vi "数据查询_数据查询_古田户外.vi"() -> ()   [LabVIEW 2016]
uses:
  <vilib>/Utility/miscctls.llb/LVPointTypeDef.ctl
  <vilib>/Utility/miscctls.llb/LVRowAndColumnUnsignedTypeDef.ctl
  <vilib>/addons/database/_DB Variant To Data/Database Variant To Data.xnode
panel:
  in  "工作模式":string(combo)="全部数据"
  out "连接的字符串":string
  out "选中数据表":string
  in  "查询":bool
  in  "结束日期":string="2020/01/01"
  in  "起始日期":string="2010/01/01"
  out "XY图":cluster{"data":timestamp[], "data":dbl[]}[](graph)
  in  "组合框":string(combo)
  out "数据表":string[][](table)
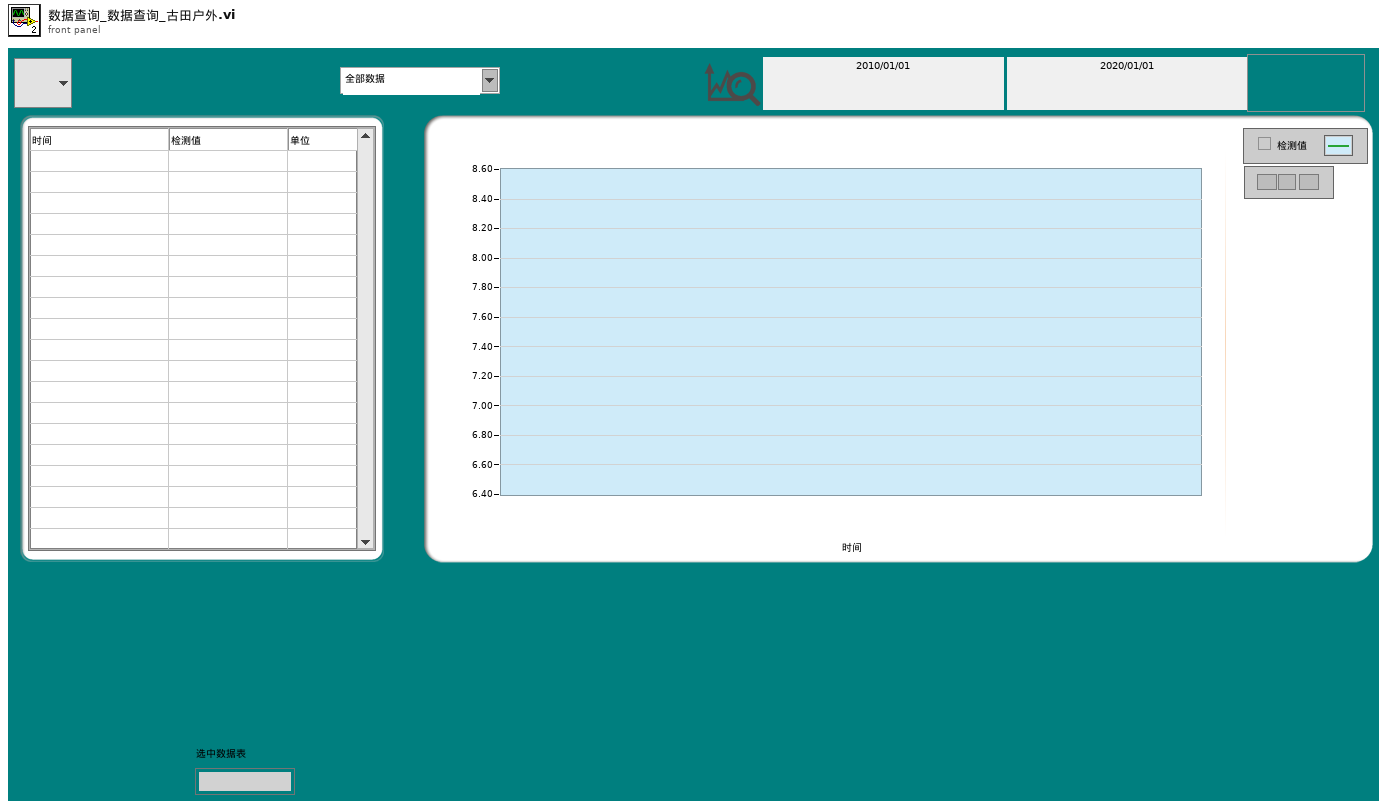
[diagram p1: front panel]
types:
  T1 = typedef "LVPointTypeDef.ctl" = cluster{"Horizontal":i16, "Vertical":i16}
  T2 = typedef "LVRowAndColumnUnsignedTypeDef.ctl" = cluster{"Row":u32, "Column":u32}
  T3 = typedef "LVPoint32TypeDef.ctl" = cluster{"Horizontal":i32, "Vertical":i32}
  T4 = typedef "LVPointDoubleTypeDef.ctl" = cluster{"Cursor X":dbl, "Cursor Y":dbl}
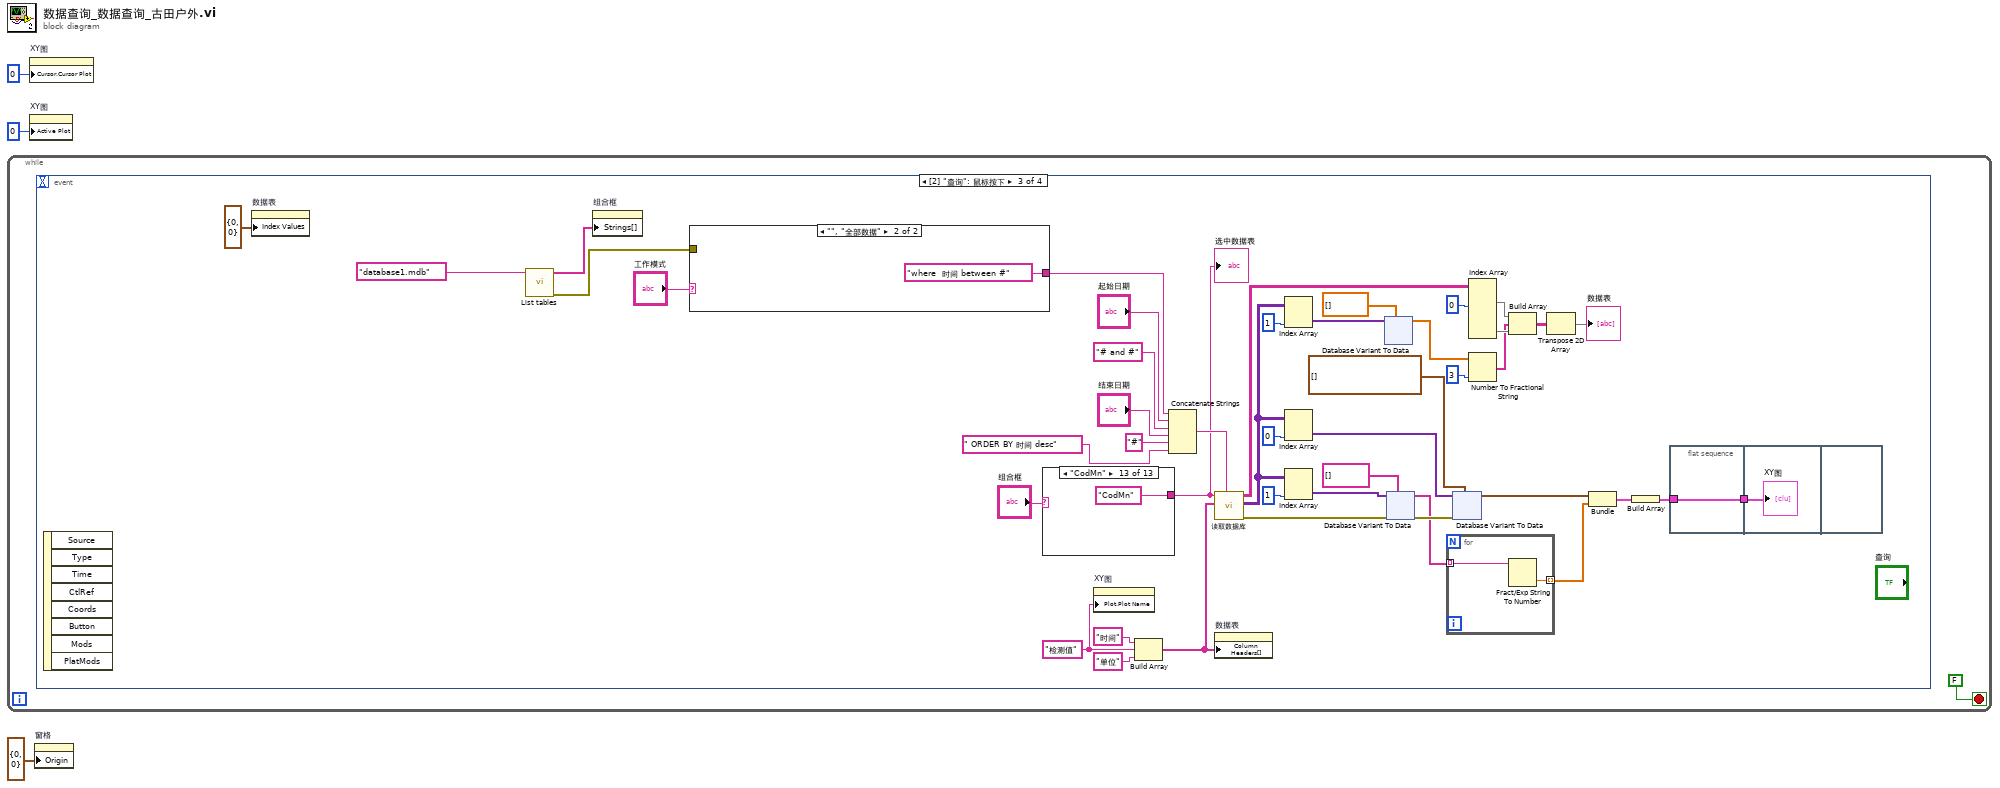
[diagram p0: block diagram]
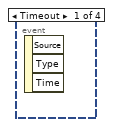
[diagram p2: hidden frame]
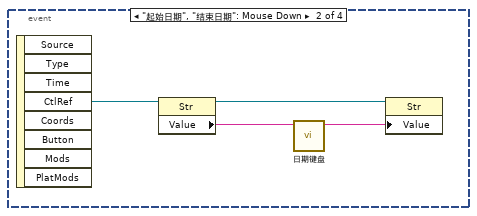
[diagram p3: hidden frame]
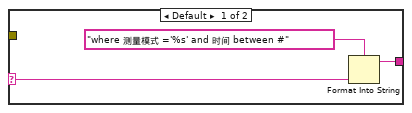
[diagram p4: hidden frame]
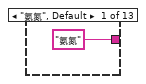
[diagram p5: hidden frame]
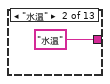
[diagram p6: hidden frame]
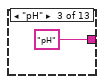
[diagram p7: hidden frame]
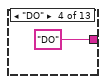
[diagram p8: hidden frame]
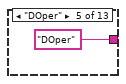
[diagram p9: hidden frame]
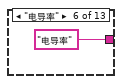
[diagram p10: hidden frame]
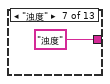
[diagram p11: hidden frame]
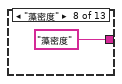
[diagram p12: hidden frame]
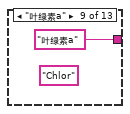
[diagram p13: hidden frame]
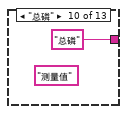
[diagram p14: hidden frame]
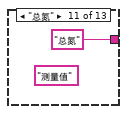
[diagram p15: hidden frame]
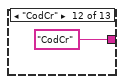
[diagram p16: hidden frame]
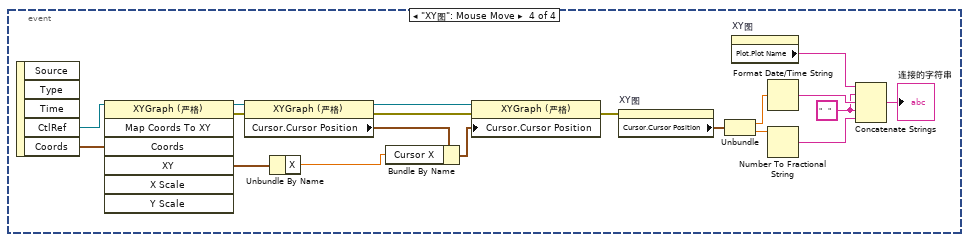
[diagram p17: hidden frame]
diagram:
  n1 = while {
    stop <- FALSE stop-if-true
    n2 = event shown="[2] \"查询\": 鼠标按下" {
      selector: _ -> [_ _ _ _]
      dyn-events: _ -> [_ _ _ _]
      timeout: _ -> [_ _ _ _]
      event Timeout {
        n3 = event-data() -> ()  [unwired: 1 in, 3 out]
      }
      event "起始日期", "结束日期": Mouse Down {
        n4 = event-data() -> ("CtlRef"=w8:refnum<vi>)  [unwired: 1 in, 7 out]
        n5 = property class="Str"(reference=w8) -> (reference out=w6:refnum<vi>, "Value"=w7:string)  [unwired: 1 in, 1 out]
        n6 = call "日期键盘.vi"("原值"=w7) -> ("x+y"=w5:string)  [unwired: 10 in]
        n7 = property class="Str"(reference=w6, "Value"=w5) -> ()  [unwired: 1 in, 2 out]
      }
      event "查询": Mouse Down {
        w25 = "检测值"
        n8 = event-data() -> ()  [unwired: 1 in, 8 out]
        n9 = property on="数据表" class="Tbl (严格)"("Index Values"=T2 {"Row"=0, "Column"=0} ("索引值")) -> ()  [unwired: 2 in, 2 out]
        n10 = call "List tables.vi"("database"="database1.mdb") -> ("error out"=w9:errorcluster, "tables"=w10:string[])  [unwired: 9 in]
        n11 = property on="组合框" class="CmbBox"("Strings[]"=w10) -> ()  [unwired: 2 in, 2 out]
        n12 = case shown="\"\", \"全部数据\"" "工作模式" {
          selector: "工作模式" -> [w56 _]
          tunnel: [w54 "where  时间 between #" ("condition")] -> w13
          tunnel: w9 -> [_ _]
          frame Default {
            n13 = Format Into String(format string="where 测量模式 ='%s' and 时间 between #" ("condition"), w56) -> (resulting string=w54:string)  [unwired: 2 in, 1 out]
          }
          frame "", "全部数据" {
          }
        }
        n14 = case shown="\"CodMn\"" "组合框" {
          tunnel: ["氨氮" "水温" "pH" "DO" "DOper" "电导率" "浊度" "藻密度" "叶绿素a" "总磷" "总氮" "CodCr" "CodMn"] -> w27
          frame "氨氮", Default {
          }
          frame "水温" {
          }
          frame "pH" {
          }
          frame "DO" {
          }
          frame "DOper" {
          }
          frame "电导率" {
          }
          frame "浊度" {
          }
          frame "藻密度" {
          }
          frame "叶绿素a" {
            (unwired) "Chlor"
          }
          frame "总磷" {
            (unwired) "测量值"
          }
          frame "总氮" {
            (unwired) "测量值"
          }
          frame "CodCr" {
          }
          frame "CodMn" {
          }
        }
        "选中数据表" <- w27
        n15 = property on="XY图" class="XYGraph (严格)"("Plot.Plot Name"=w25) -> ()  [unwired: 2 in, 2 out]
        n16 = Build Array("时间", w25, "单位" ("元素")) -> (w28:string[])
        n17 = Concatenate Strings(w13, "起始日期", "# and #" ("condition"), "结束日期", "#" ("condition"), " ORDER BY 时间 desc" ("字符串")) -> (w52:string)
        n18 = call "读取数据库.vi"("condition"=w52, "显示项"=w28, "组合框"=w27) -> ("error out"=w43:errorcluster, "data"=w22:variant[][], "表格"=w35:string[][])  [unwired: 5 in, 1 out]
        n19 = property on="数据表" class="Tbl (严格)"("Column Headers[]"=w28) -> ()  [unwired: 2 in, 2 out]
        n20 = Index Array(array=w22, index (col)=1 ("禁用的索引 (列)")) -> (element=w20:variant[])  [unwired: 1 in]
        n21 = Index Array(array=w22, index (col)=0 ("禁用的索引 (列)")) -> (element=w46:variant[])  [unwired: 1 in]
        n22 = Index Array(array=w22, index (col)=1 ("禁用的索引 (列)")) -> (element=w44:variant[])  [unwired: 1 in]
        n23 = xnode "Database Variant To Data"("database variant"=w20, "type"=sgl[] []) -> ("data"=w18:sgl[])  [unwired: 1 in, 1 out]
        n24 = xnode "Database Variant To Data"("database variant"=w44, "error in (no error)"=w43, "type"=string[] []) -> ("data"=w26:string[], "error out"=w42:errorcluster)
        n25 = for {
          tunnel: w26 -> [w97] mode=indexing
          tunnel: [w96] -> w12 mode=indexing
          n26 = Fract/Exp String To Number(string=w97) -> (number=w96:dbl)  [unwired: 3 in, 1 out]
        }
        n27 = xnode "Database Variant To Data"("database variant"=w46, "error in (no error)"=w42, "type"=timestamp[] []) -> ("data"=w37:timestamp[])  [unwired: 1 out]
        n28 = Index Array(array=w35, index (col) #1=0 ("禁用的索引 (列)")) -> (element #1=w33:string[], element #3=w23:string[])  [unwired: 5 in, 1 out]
        n29 = Number To Fractional String(number=w18, precision (6)=i16 3 ("精度(6)")) -> (F-format string=w16:string[])  [unwired: 2 in]
        n30 = Build Array(w33, w16, w23) -> (w32:string[][])
        n31 = Transpose 2D Array(2D array=w32) -> (transposed array=→"数据表":string[][])
        n32 = Bundle("data"=w37, w12) -> (w38:cluster{"data":timestamp[], dbl[]})  [unwired: 1 in]
        n33 = Build Array(w38) -> (w39:cluster{"data":timestamp[], dbl[]}[])
        n34 = flat-sequence {
          tunnel: [w111] -> w40
          tunnel: w39 -> [w111]
          tunnel: w40 -> [w112]
          frame #0 {
          }
          frame #1 {
            "XY图" <- w112
          }
          frame #2 {
          }
        }
      }
      event "XY图": Mouse Move {
        w214 = "   " ("字符串")
        n35 = event-data() -> ("CtlRef"=w221:refnum<vi>, "Coords"=w220:T3)  [unwired: 1 in, 3 out]
        n36 = invoke class="XYGraph (严格)" method="Map Coords To XY"(reference=w221, "Coords"=w220) -> (reference out=w209:refnum<vi>, error out=w207:errorcluster, "XY"=w210:cluster{"X":dbl, "Y":dbl})  [unwired: 5 in, 4 out]
        n37 = property class="XYGraph (严格)"(reference=w209, error in=w207) -> (reference out=w208:refnum<vi>, error out=w206:errorcluster, "Cursor.Cursor Position"=w205:T4)
        n38 = Unbundle By Name(w210) -> ("X"=w204:dbl)
        n39 = Bundle By Name(cluster=w205, "Cursor X"=w204) -> (w203:T4)
        n40 = property class="XYGraph (严格)"(reference=w208, error in=w206, "Cursor.Cursor Position"=w203) -> (error out=w219:errorcluster)  [unwired: 1 out]
        n41 = property on="XY图" class="XYGraph (严格)"(error in=w219) -> ("Cursor.Cursor Position"=w217:T4)  [unwired: 1 in, 2 out]
        n42 = Unbundle(w217) -> ("Cursor X"=w216:dbl, "Cursor Y"=w213:dbl)
        n43 = property on="XY图" class="XYGraph (严格)"() -> ("Plot.Plot Name"=w211:string)  [unwired: 2 in, 2 out]
        n44 = Format Date/Time String(seconds (now)=w216) -> (date/time string=w215:string)  [unwired: 2 in]
        n45 = Number To Fractional String(number=w213) -> (F-format string=w212:string)  [unwired: 3 in]
        n46 = Concatenate Strings(w211, w214, w215, w214, w212) -> (→"连接的字符串":string)
      }
    }
  }
  n47 = property on="XY图" class="XYGraph (严格)"("Cursor.Cursor Plot"=0 ("游标.游标关联曲线")) -> ()  [unwired: 2 in, 2 out]
  n48 = property on="XY图" class="XYGraph (严格)"("Active Plot"=u32 0 ("活动曲线")) -> ()  [unwired: 2 in, 2 out]
  n49 = property on="窗格" class="Pane"("Origin"=T1 {"Horizontal"=0, "Vertical"=0} ("原点")) -> ()  [unwired: 2 in, 2 out]
